vi "String to Controller Type.vi"(11 "String":string) -> (3 "Controller Type":T1)   [LabVIEW 2020, in "Generic Plugin.lvclass"]
uses:
  Generic Plugin.lvclass
  Controller Type.ctl
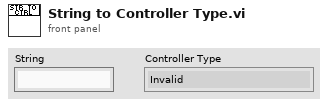
[diagram p1: front panel]
types:
  T1 = typedef "Generic Plugin.lvclass/Controller Type.ctl" = enum16{"Invalid", "Temperature Controller", "Pump Controller", "Generic Optimizer", "LC Parser"}
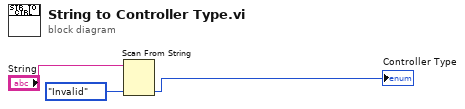
[diagram p0: block diagram]
diagram:
  n1 = Scan From String(input string="String", default 1=Controller_Type."Invalid" ("Controller Type")) -> (output 1=→"Controller Type":T1)  [unwired: 3 in, 3 out]
